vi "auto_modNL.vi"() -> ()   [LabVIEW 2012, in "BlockParty4150.lvrbt"]
uses:
  BlockParty4150.lvrbt
  <vilib>/NXT/Subs/LVHSConnector.ctl
  <vilib>/NXT/LegoClasses/BrickReference/BrickReference.lvclass
  <vilib>/NXT/Hardware/Plugins/Tetrix 180 deg Servo/Tetrix180ServoAddress.ctl
  <vilib>/NXT/Hardware/Plugins/Tetrix DC Motor/TetrixDCMotorAddress.ctl
  <vilib>/NXT/HiTechnic/HiTechnic Controls/HiTechnic Port.ctl
  <vilib>/NXT/Block Support/NXT_InputPort.ctl
  <vilib>/NXT/Dual Mode Library/Display/drawText.vi
  <vilib>/NXT/Dual Mode Library/Sound/Tone.vi
  <vilib>/NXT/NXTIO Xnodes/NXTIONodeSubVIs/TETRIX IO Move DC Motors.vi
  <vilib>/NXT/NXTIO Xnodes/NXTIONodeSubVIs/TETRIX IO Stop DC Motors.vi
  <vilib>/NXT/NXTIO Xnodes/NXTIONodeSubVIs/TETRIX IO Move Servos.vi
  <vilib>/NXT/Dual Mode Library/Waits/Wait_Num(msec).vi
  <vilib>/NXT/NXTIO Xnodes/AddressXNode/NXTIOAddress.xnode
  <vilib>/NXT/NXTIO Xnodes/NXTIOXNode/NXTIO.xnode
panel:
  out "Enabled":bool
  out "iter":i32
  out "NXT":T1
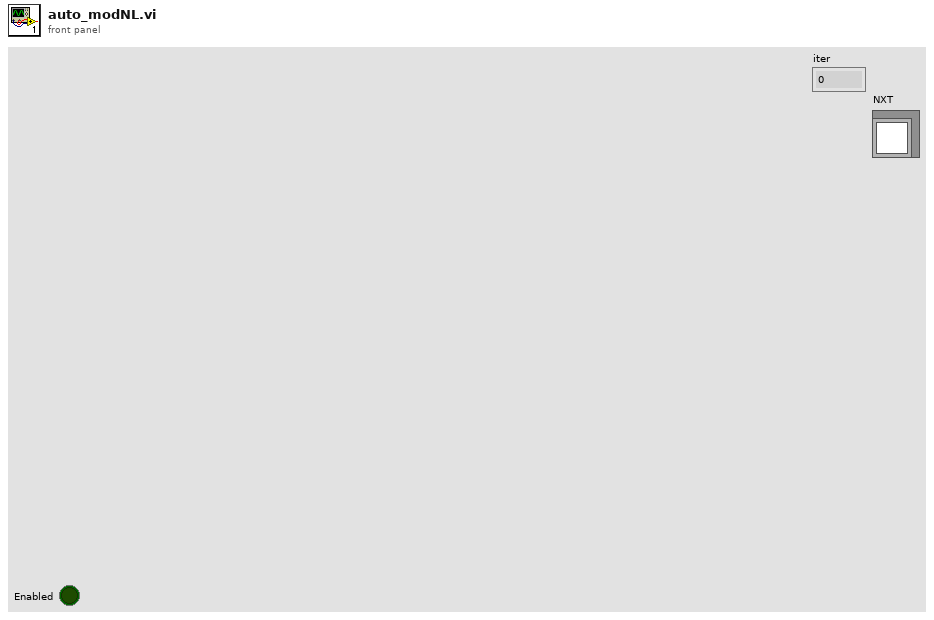
[diagram p1: front panel]
types:
  T1 = typedef "LVHSConnector.ctl" = refnum<class "BrickReference.lvclass">
  T2 = typedef "Tetrix180ServoAddress.ctl" = i16
  T3 = typedef "TetrixDCMotorAddress.ctl" = i16
  T4 = typedef "HiTechnic Port.ctl" = cluster{"Port":T5, "MUX Port":u8}
  T5 = typedef "NXT_InputPort.ctl" = u8
  T6 = cluster{"Direction (0-9)":i16, "Signal Strength (Array)":u8[]}
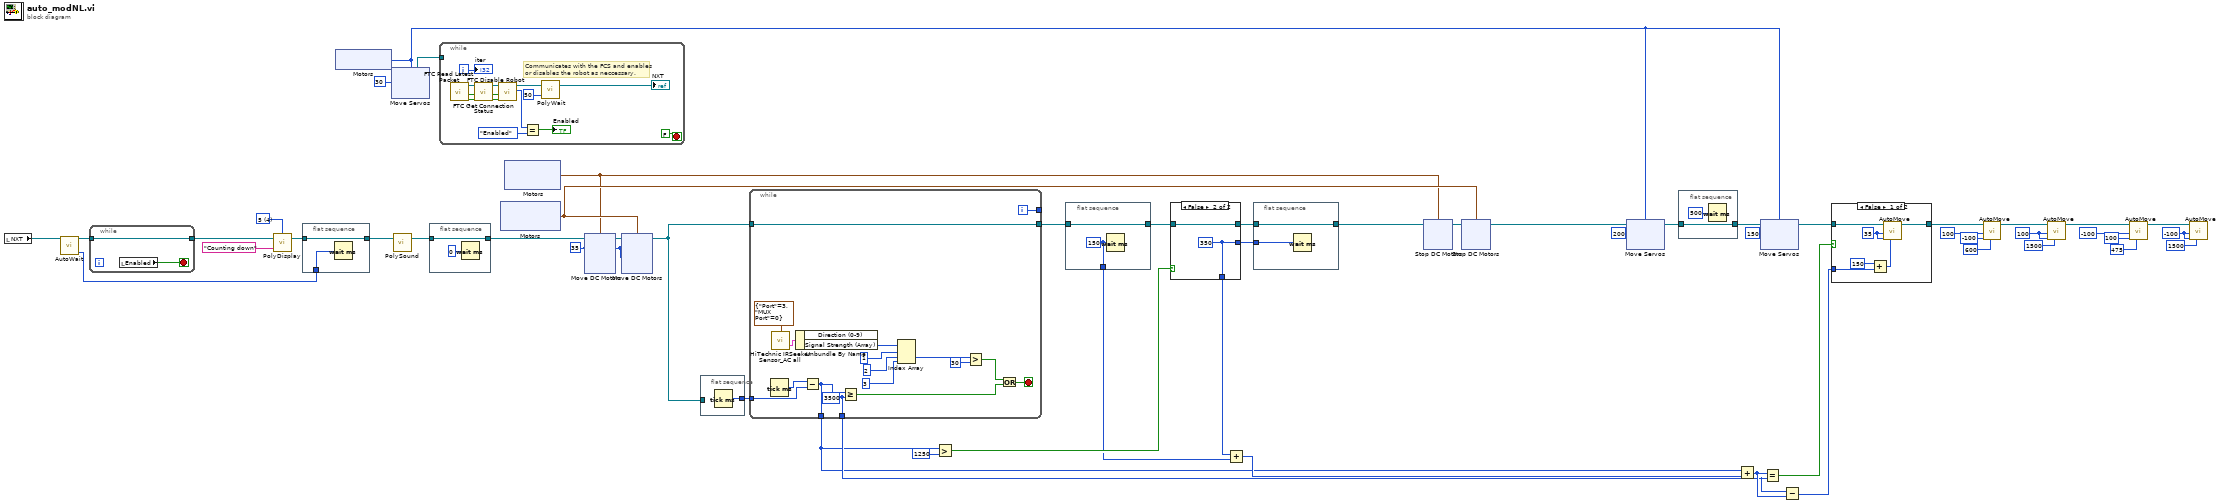
[diagram p0: block diagram]
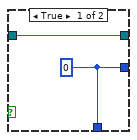
[diagram p3: hidden frame]
diagram:
  w14 = i8 -100 ("Left Power")
  w19 = i8 100 ("Left Power")
  w28 = i16 4 items=["1", "2", "3", "4", "5", "6", "7", "8"] ("Line")
  w50 = i8 35 ("Power/Speed 1")
  n1 = local read "NXT"() -> (w52:T1)
  n2 = call "AutoWait.vi"("BrickReference in"=w52) -> ("TimeDelay"=w25:u32, "BrickReference out"=w24:T1)  [unwired: 9 in]
  n3 = while {
    tunnel: [w57] -> w23
    tunnel: w24 -> [w57]
    stop <- w56 stop-if-true
    n4 = local read "Enabled"() -> (w56:bool)
  }
  n5 = call-poly <vilib>:"PolyDisplay.vi"("Text"="Counting down", "NXT"=w23, "Line"=w28) -> ("NXT"=w30:T1)  [unwired: 1 in]
  n6 = flat-sequence {
    tunnel: w30 -> [w59]
    tunnel: [w59] -> w27
    tunnel: w25 -> [w58]
    frame #0 {
      n7 = Wait (ms)(milliseconds to wait=w58) -> ()  [unwired: 1 out]
    }
  }
  n8 = xnode "Motors"() -> ("Motor"=w53:T2)
  n9 = xnode "Move Servos"("Position 1"=u8 30, "Servos"=w53) -> ("NXT"=w54:T1)  [unwired: 1 in]
  n10 = call-poly <vilib>:"PolySound.vi"("NXT"=w27) -> ("NXT"=w26:T1)  [unwired: 3 in]
  n11 = flat-sequence {
    tunnel: w26 -> [w61]
    tunnel: [w61] -> w47
    frame #0 {
      n12 = Wait (ms)(milliseconds to wait=u32 0) -> ()  [unwired: 1 out]
    }
  }
  n13 = while {
    tunnel: w54 -> [_]
    i -> [w63]
    stop <- FALSE stop-if-true
    # "Communicates with the FCS and enables \nor disables the robot as neccessary."
    n14 = call <vilib>:"FTC Read Latest Packet.vi"() -> ("Packet Received?"=w73:bool, "Stopped?"=w72:bool, "NXT"=w75:T1)  [unwired: 6 in, 3 out]
    n15 = call <vilib>:"FTC Get Connection Status.vi"("Packet Received?"=w73, "Stopped?"=w72, "NXT"=w75) -> ("Online?"=w65:bool, "Stopped?"=w66:bool, "NXT"=w74:T1)  [unwired: 5 in]
    n16 = call <vilib>:"FTC Disable Robot.vi"("Online?"=w65, "Stopped?"=w66, "NXT"=w74) -> ("Enabled?"=w69:enum16{"Disabled", "Enabled"}, "NXT"=w71:T1)  [unwired: 3 in]
    n17 = Equal?(x=w69, y=enum16{"Disabled", "Enabled"}."Enabled") -> (x = y?=→"Enabled":bool)
    n18 = call-poly <vilib>:"PolyWait.vi"("Time (100 msec)"=u32 50 ("Time (msec)"), "NXT"=w71) -> ("NXT"=→"NXT":T1)  [unwired: 2 in]
    "iter" <- w63
  }
  n19 = xnode "Motors"() -> ("Motor"=w9:cluster{"TetrixDCMotor":T3, "TetrixDCMotor":T3})
  n20 = xnode "Motors"() -> ("Motor"=w1:cluster{"TetrixDCMotor":T3, "TetrixDCMotor":T3})
  n21 = xnode "Move DC Motors"("Power/Speed 2"=w50, "Power/Speed 1"=w50, "Motors"=w1, "NXT"=w47) -> ("NXT"=w51:T1)
  n22 = xnode "Move DC Motors"("Power/Speed 2"=w50, "Power/Speed 1"=w50, "Motors"=w9, "NXT"=w51) -> ("NXT"=w48:T1)
  n23 = flat-sequence {
    tunnel: [w76] -> w46
    tunnel: w48 -> [_]
    frame #0 {
      n24 = Tick Count (ms)() -> (millisecond timer value=w76:u32)
    }
  }
  n25 = while {
    tunnel: [w92] -> _
    tunnel: w48 -> [w85]
    tunnel: [w85] -> w45
    tunnel: w46 -> [w79]
    tunnel: [w78] -> w31
    tunnel: [w77] -> w37
    i -> [w92]
    stop <- w83 stop-if-true
    w77 = u32 3500 ("y")
    n26 = Tick Count (ms)() -> (millisecond timer value=w93:u32)
    n27 = call <vilib>:"HiTechnic IRSeeker Sensor_AC all.vi"("Port/MUX"=T4 {"Port"=3, "MUX Port"=0}) -> ("All Info"=w91:T6)  [unwired: 2 in, 1 out]
    n28 = Unbundle By Name(w91) -> ("Signal Strength (Array)"=w90:u8[])  [unwired: 1 out]
    n29 = Subtract(x=w93, y=w79) -> (x-y=w78:u32)
    n30 = Greater Or Equal?(x=w78, y=w77) -> (x >= y?=w81:bool)
    n31 = Index Array(array=w90, index #1=1 ("index"), index #2=2 ("index"), index #3=3 ("index")) -> (element #2=w80:u8)  [unwired: 2 out]
    n32 = Greater?(x=w80, y=u8 30) -> (0:w82:bool)
    n33 = Or(x=w82, y=w81) -> (x .or. y?=w83:bool)
  }
  n34 = Greater?(x=w31, y=u32 1250) -> (0:w35:bool)
  n35 = flat-sequence {
    tunnel: [w95] -> w38
    tunnel: w45 -> [w95]
    tunnel: [w94] -> w32
    frame #0 {
      w94 = u32 150 ("milliseconds to wait")
      n36 = Wait (ms)(milliseconds to wait=w94) -> ()  [unwired: 1 out]
    }
  }
  n37 = case shown="False" w35 {
    tunnel: w38 -> [w96 w98]
    tunnel: [w96 w98] -> w8
    tunnel: [w97 w99] -> w34
    tunnel: [w97 w99] -> w7
    frame True {
      w97 = u32 0 ("milliseconds to wait")
    }
    frame False {
      w99 = u32 350 ("milliseconds to wait")
    }
  }
  n38 = Add(x=w34, y=w32) -> (x+y=w33:u32)
  n39 = flat-sequence {
    tunnel: [w101] -> w6
    tunnel: w8 -> [w101]
    tunnel: w7 -> [w100]
    frame #0 {
      n40 = Wait (ms)(milliseconds to wait=w100) -> ()  [unwired: 1 out]
    }
  }
  n41 = xnode "Stop DC Motors"("Motors"=w1, "NXT"=w6) -> ("NXT"=w49:T1)
  n42 = xnode "Stop DC Motors"("Motors"=w9, "NXT"=w49) -> ("NXT"=w40:T1)
  n43 = xnode "Move Servos"("Position 1"=u8 200, "Servos"=w53, "NXT"=w40) -> ("NXT"=w43:T1)
  n44 = flat-sequence {
    tunnel: [w102] -> w41
    tunnel: w43 -> [w102]
    frame #0 {
      n45 = Wait (ms)(milliseconds to wait=u32 500) -> ()  [unwired: 1 out]
    }
  }
  n46 = Add(x=w31, y=w33) -> (x+y=w39:u32)
  n47 = xnode "Move Servos"("Position 1"=u8 150, "Servos"=w53, "NXT"=w41) -> ("NXT"=w3:T1)
  n48 = Equal?(x=w39, y=w37) -> (x = y?=w4:bool)
  n49 = Subtract(x=w37, y=w39) -> (x-y=w5:u32)
  n50 = case shown="False" w4 {
    tunnel: w5 -> [w106 _]
    tunnel: [w104 w110] -> w2
    tunnel: w3 -> [w105 w110]
    frame False {
      w109 = i8 35 ("Left Power")
      n51 = Add(x=u32 150, y=w106) -> (x+y=w107:u32)
      n52 = call "AutoMove.vi"("Wait"=w107, "Right Power"=w109, "Left Power"=w109, "BrickReference in"=w105) -> ("BrickReference out"=w104:T1)  [unwired: 7 in]
    }
    frame True {
    }
  }
  n53 = call "AutoMove.vi"("Wait"=u32 600, "Right Power"=i8 -100, "Left Power"=i8 100, "BrickReference in"=w2) -> ("BrickReference out"=w10:T1)  [unwired: 7 in]
  n54 = call "AutoMove.vi"("Wait"=u32 1500, "Right Power"=w19, "Left Power"=w19, "BrickReference in"=w10) -> ("BrickReference out"=w12:T1)  [unwired: 7 in]
  n55 = call "AutoMove.vi"("Wait"=u32 475, "Right Power"=i8 100, "Left Power"=i8 -100, "BrickReference in"=w12) -> ("BrickReference out"=w11:T1)  [unwired: 7 in]
  n56 = call "AutoMove.vi"("Wait"=u32 1500, "Right Power"=w14, "Left Power"=w14, "BrickReference in"=w11) -> ()  [unwired: 7 in, 1 out]
